vi "registerForEvent.vi"(8 "error in (no error)":errorcluster, 11 "Event in":refnum<class "Event.lvclass">) -> (0 "error out":errorcluster, 1 "Event":refnum<user-event>, 2 "Event Registration Refnum":refnum<event-registration>, 3 "Event out":refnum<class "Event.lvclass">)   [LabVIEW 2009, in "Events.lvlib" / "Event.lvclass"]
uses:
  Event.lvclass
  Event.lvclass/Event.ctl
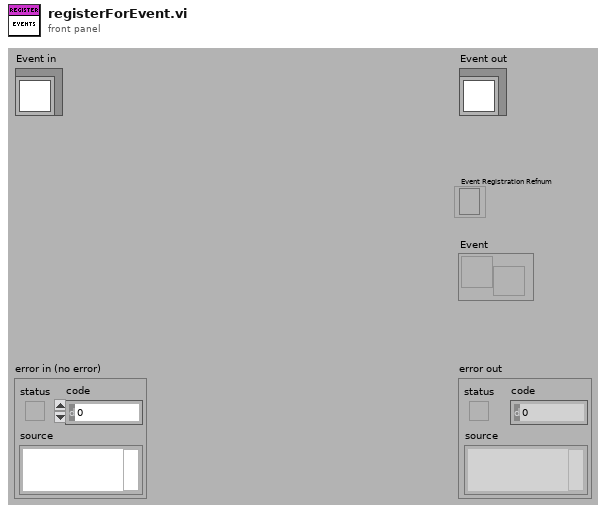
[diagram p1: front panel]
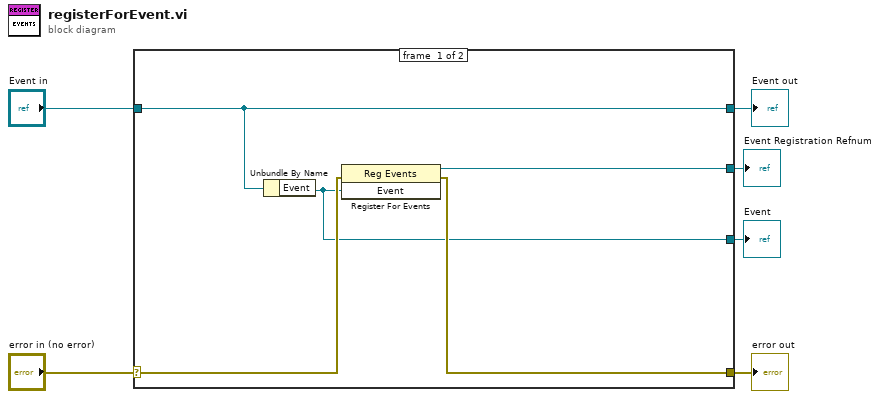
[diagram p0: block diagram]
diagram:
  n1 = case shown="No Error" "error in (no error)" {
    selector: "error in (no error)" -> [w10 w13]
    tunnel: [w9 w13] -> w5
    tunnel: [w11 w12] -> w3
    tunnel: "Event in" -> [w11 w12]
    tunnel: [w8 _] -> w2
    tunnel: [w7 _] -> w1
    frame #0 {
      n2 = Unbundle By Name(w11) -> ("Event"=w7:refnum<user-event>)
      n3 = register-events(error in=w10, w7) -> (reference out=w8:refnum<event-registration>, error out=w9:errorcluster)  [unwired: 1 in]
    }
    frame #1 {
    }
  }
  "error out" <- w5
  "Event out" <- w3
  "Event Registration Refnum" <- w2
  "Event" <- w1
